vi "Dispatch Message.vi"(8 "error in":errorcluster, 11 "Message":T1) -> (0 "error out":errorcluster, 3 "queue name":string)   [LabVIEW 2021]
uses:
  Message.ctl
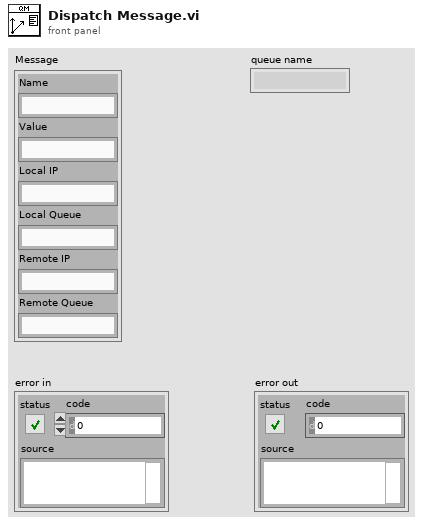
[diagram p1: front panel]
types:
  T1 = typedef "Message.ctl" = cluster{"Name":string, "Value":string, "Local IP":string, "Local Queue":string, "Remote IP":string, "Remote Queue":string}
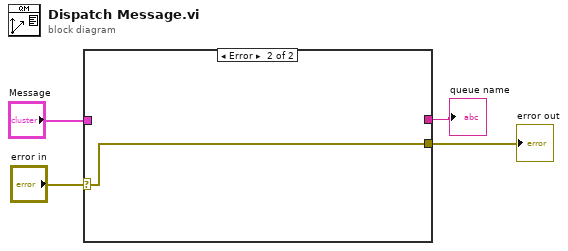
[diagram p0: block diagram]
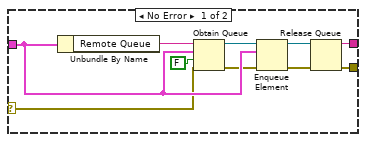
[diagram p2: hidden frame]
diagram:
  n1 = case shown="Error" "error in" {
    selector: "error in" -> [w5 w15]
    tunnel: "Message" -> [w12 _]
    tunnel: [w7 w15] -> w3
    tunnel: [w6 _] -> w2
    frame No Error {
      n2 = Unbundle By Name(w12) -> ("Remote Queue"=w14:string)
      n3 = Obtain Queue(name (unnamed)=w14, element data type=w12, create if not found? (T)=FALSE, error in (no error)=w5) -> (queue out=w13:refnum<queue>, error out=w11:errorcluster)  [unwired: 1 in, 1 out]
      n4 = Enqueue Element(queue=w13, element=w12, error in (no error)=w11) -> (queue out=w8:refnum<queue>, error out=w9:errorcluster)  [unwired: 1 in, 1 out]
      n5 = Release Queue(queue=w8, error in (no error)=w9) -> (queue name=w6:string, error out=w7:errorcluster)  [unwired: 1 in, 1 out]
    }
    frame Error {
    }
  }
  "error out" <- w3
  "queue name" <- w2
